vi "List And Filter Controls From VI.vi"(8 "Error In":errorcluster, 11 "VI Refnum":refnum<vi>) -> (0 "Error Out":errorcluster, 3 "Control Sets":T1)   [LabVIEW 2021, in "Appearance Actor.lvlib" / "Generic Theme.lvclass"]
uses:
  Generic Theme.lvclass
  Typedefs/Control Reference Lists--cluster.ctl
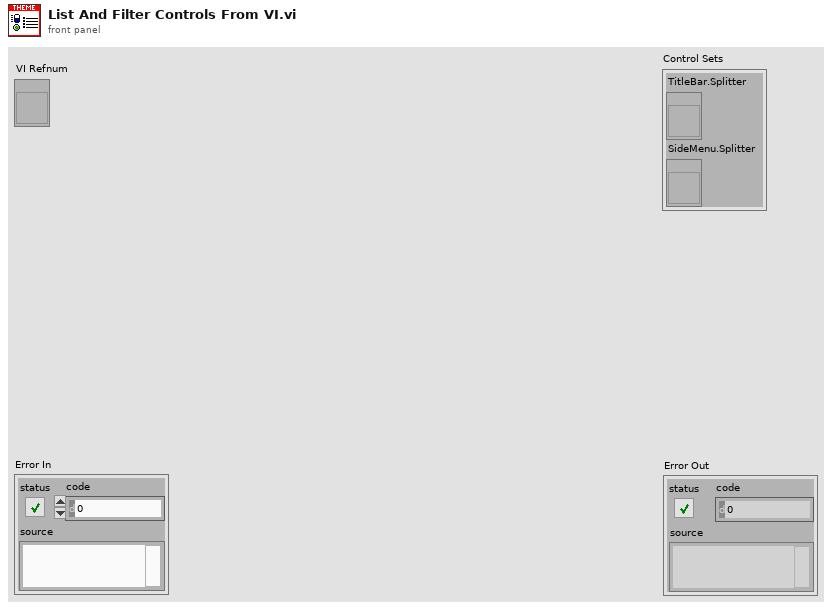
[diagram p1: front panel]
types:
  T1 = typedef "Appearance Actor.lvlib/Generic Theme.lvclass/Control Reference Lists--cluster.ctl" = cluster{"TitleBar.Splitter":refnum<vi>, "SideMenu.Splitter":refnum<vi>}
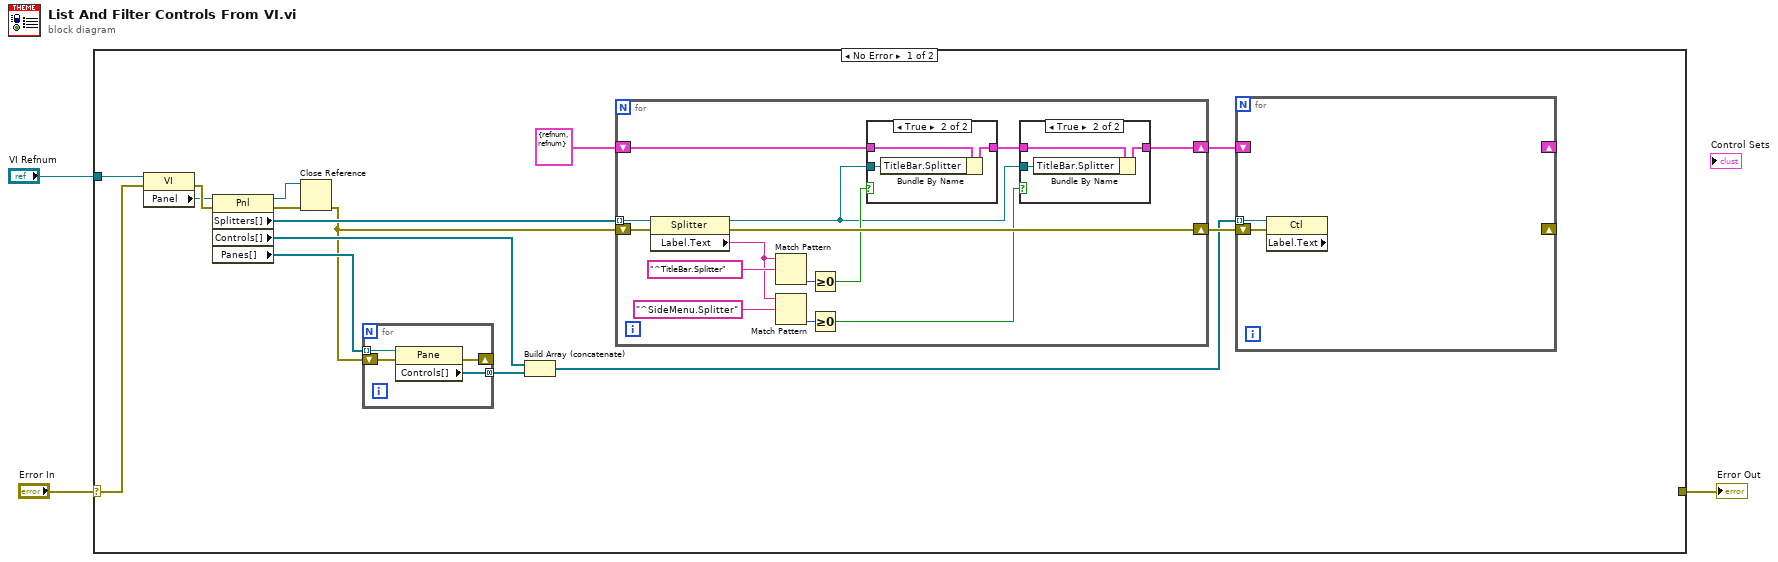
[diagram p0: block diagram]
diagram:
  n1 = case shown="No Error" "Error In" {
    selector: "Error In" -> [w16 w47]
    tunnel: "VI Refnum" -> [w18 _]
    tunnel: [_ w47] -> w1
    frame No Error {
      n2 = property class="VI"(reference=w18, error in=w16) -> (error out=w15:errorcluster, "Panel"=w14:refnum<vi>)  [unwired: 1 out]
      n3 = property class="Pnl"(reference=w14, error in=w15) -> (reference out=w17:refnum<vi>, error out=w10:errorcluster, "Splitters[]"=w9:refnum<vi>[], "Controls[]"=w12:refnum<vi>[], "Panes[]"=w13:refnum<vi>[])
      n4 = Close Reference(reference=w17, error in (no error)=w10) -> (error out=w8:errorcluster)
      n5 = for {
        tunnel: w13 -> [w46] mode=indexing
        shift-right: [w44] -> _
        shift-left: w8 -> [w45]
        tunnel: [w43] -> w11 mode=concatenating
        n6 = property class="Pane"(reference=w46, error in=w45) -> (error out=w44:errorcluster, "Controls[]"=w43:refnum<vi>[])  [unwired: 1 out]
      }
      n7 = Build Array (concatenate)(w12, w11) -> (w4:refnum<vi>[])
      n8 = for {
        tunnel: w9 -> [w34] mode=indexing
        shift-right: [w32] -> w5
        shift-left: w8 -> [w33]
        shift-right: [w23] -> w6
        shift-left: T1 {"TitleBar.Splitter"=refnum, "SideMenu.Splitter"=refnum} ("Control Reference Lists") -> [w26]
        n9 = property class="Splitter"(reference=w34, error in=w33) -> (reference out=w21:refnum<vi>, error out=w32:errorcluster, "Label.Text"=w27:string)
        n10 = Match Pattern(string=w27, regular expression="^TitleBar.Splitter") -> (offset past match=w30:i32)  [unwired: 1 in, 3 out]
        n11 = Match Pattern(string=w27, regular expression="^SideMenu.Splitter") -> (offset past match=w29:i32)  [unwired: 1 in, 3 out]
        n12 = Greater Or Equal To 0?(x=w30) -> (x >= 0?=w25:bool)
        n13 = Greater Or Equal To 0?(x=w29) -> (x >= 0?=w22:bool)
        n14 = case shown="True" w25 {
          tunnel: w26 -> [w39 w42]
          tunnel: [w39 w41] -> w24
          tunnel: w21 -> [_ w40]
          frame False {
          }
          frame True {
            n15 = Bundle By Name(cluster=w42, "TitleBar.Splitter"=w40) -> (w41:T1)
          }
        }
        n16 = case shown="True" w22 {
          tunnel: w24 -> [w35 w38]
          tunnel: [w35 w37] -> w23
          tunnel: w21 -> [_ w36]
          frame False {
          }
          frame True {
            n17 = Bundle By Name(cluster=w38, "TitleBar.Splitter"=w36) -> (w37:T1)
          }
        }
      }
      n18 = for {
        shift-right: _ -> [_]
        shift-left: w6 -> [_]
        shift-right: _ -> [_]
        shift-left: w5 -> [w19]
        tunnel: w4 -> [w20] mode=indexing
        n19 = property class="Ctl" props=["Label", "Text"](reference=w20, error in=w19) -> ()  [unwired: 3 out]
      }
    }
    frame Error {
    }
  }
  "Error Out" <- w1
